vi "BenchmarkToFile.vi"(4 "Memory":dbl, 6 "CPU":dbl, 7 "device name":string, 8 "error in (no error)":errorcluster) -> (0 "error out":errorcluster)   [LabVIEW 2017, in "Benchmarking.lvlib"]
uses:
  <vilib>/addons/InsightCM/Devices/Shared/Common/Benchmarking/Benchmarking.lvlib
  <vilib>/addons/PointValueMap/subVIs/Point_Read_double.vi
  <vilib>/addons/InsightCM/Utilities/GlobalConfiguration/GlobalConfiguration.lvlib
  <vilib>/addons/PointValueMap/PointValueMap.lvlib
  <vilib>/addons/TraceLogger/TraceLogger.lvlib
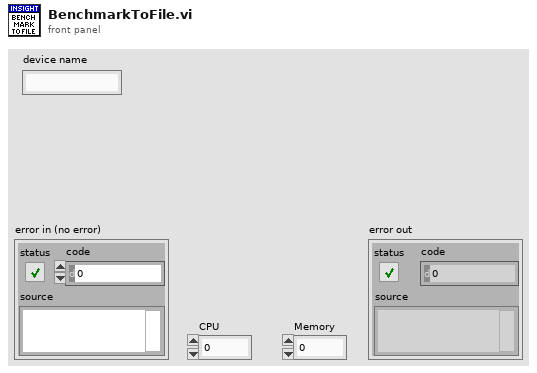
[diagram p1: front panel]
types:
  T1 = enum16{"open", "replace", "create", "open or create", "replace or create", "replace or create with confirmation"}
  T2 = typedef "PointValueMap.lvlib/PointMap.ctl" = refnum<data-value>
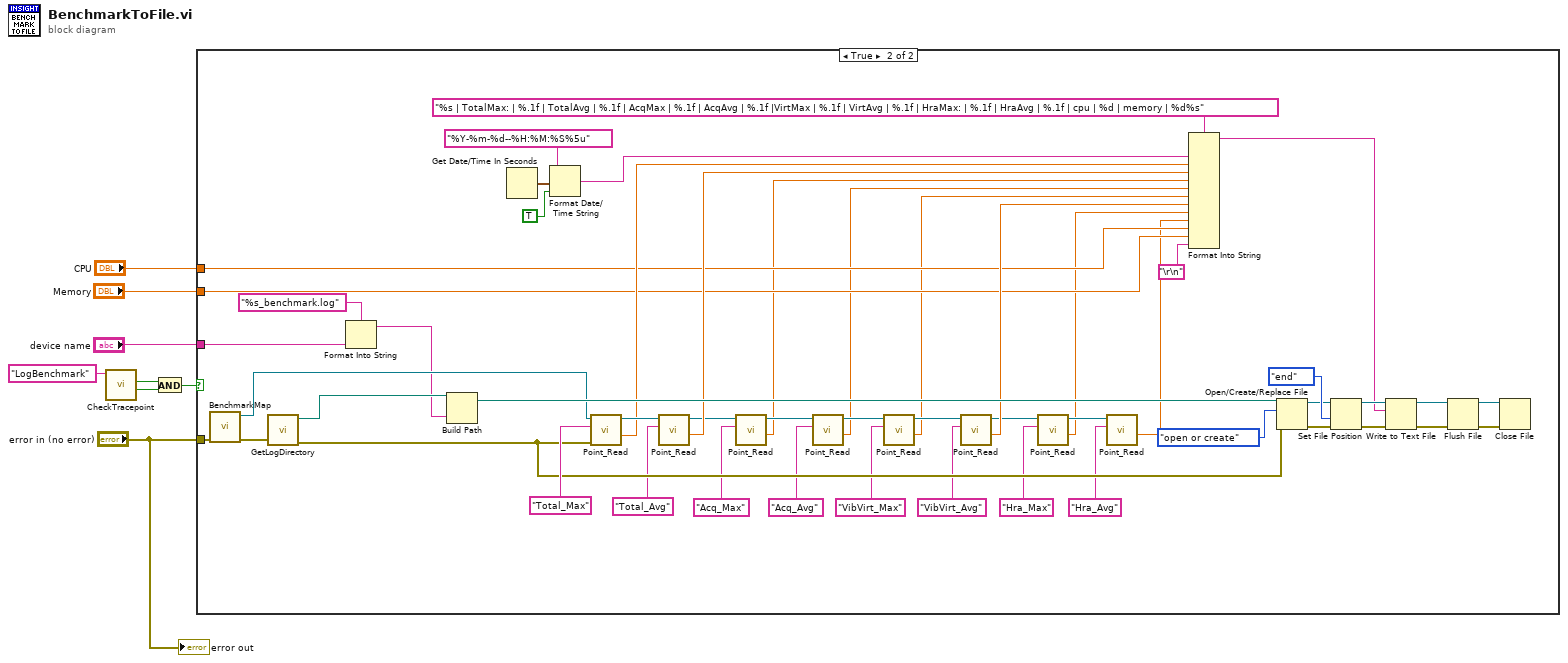
[diagram p0: block diagram]
diagram:
  n1 = call <vilib>:"CheckTracepoint.vi"("tracepoint"="LogBenchmark") -> ("found"=w3:bool, "enabled"=w2:bool)  [unwired: 8 in, 1 out]
  n2 = And(x=w2, y=w3) -> (x .and. y?=w1:bool)
  n3 = case shown="True" w1 {
    tunnel: "CPU" -> [_ w33]
    tunnel: "Memory" -> [_ w32]
    tunnel: "error in (no error)" -> [_ w24]
    tunnel: "device name" -> [_ w21]
    frame False {
    }
    frame True {
      n4 = call <vilib>:"BenchmarkMap.vi"("error in (no error)"=w24) -> ("error out"=w25:errorcluster, "benchmark map"=w23:T2)  [unwired: 9 in]
      n5 = call <vilib>:"GetLogDirectory.vi"("error in (no error)"=w25) -> ("error out"=w42:errorcluster, "log dir"=w44:path)  [unwired: 9 in]
      n6 = Format Into String(format string="%s_benchmark.log", w21) -> (resulting string=w20:string)  [unwired: 2 in, 1 out]
      n7 = Build Path(base path=w44, name or relative path=w20) -> (appended path=w43:path)
      n8 = Get Date/Time In Seconds() -> (seconds since 1Jan1904=w47:timestamp)
      n9 = Format Date/Time String(time format string (%c)="%Y-%m-%d--%H:%M:%S%5u", seconds (now)=w47, UTC format=TRUE) -> (date/time string=w10:string)
      n10 = call-poly <vilib>:"Point_Read.vi"("Error In"=w42, "Tag"="Total_Max", "Map"=w23) -> ("Value"=w38:dbl, "Map Out"=w41:T2)  [unwired: 3 in, 4 out]
      n11 = call-poly <vilib>:"Point_Read.vi"("Tag"="Total_Avg", "Map"=w41) -> ("Value"=w39:dbl, "Map Out"=w16:T2)  [unwired: 4 in, 4 out]
      n12 = call-poly <vilib>:"Point_Read.vi"("Tag"="Acq_Max", "Map"=w16) -> ("Value"=w14:dbl, "Map Out"=w17:T2)  [unwired: 4 in, 4 out]
      n13 = call-poly <vilib>:"Point_Read.vi"("Tag"="Acq_Avg", "Map"=w17) -> ("Value"=w13:dbl, "Map Out"=w15:T2)  [unwired: 4 in, 4 out]
      n14 = call-poly <vilib>:"Point_Read.vi"("Tag"="VibVirt_Max", "Map"=w15) -> ("Value"=w12:dbl, "Map Out"=w37:T2)  [unwired: 4 in, 4 out]
      n15 = call-poly <vilib>:"Point_Read.vi"("Tag"="VibVirt_Avg", "Map"=w37) -> ("Value"=w34:dbl, "Map Out"=w31:T2)  [unwired: 4 in, 4 out]
      n16 = call-poly <vilib>:"Point_Read.vi"("Tag"="Hra_Max", "Map"=w31) -> ("Value"=w27:dbl, "Map Out"=w30:T2)  [unwired: 4 in, 4 out]
      n17 = call-poly <vilib>:"Point_Read.vi"("Tag"="Hra_Avg", "Map"=w30) -> ("Value"=w26:dbl)  [unwired: 4 in, 5 out]
      n18 = Format Into String(format string="%s | TotalMax: | %.1f | TotalAvg | %.1f | AcqMax | %.1f | AcqAvg | %.1f |VirtMax | %.1f | VirtAvg | %.1f | HraMax: | %.1f | HraAvg | %.1f | cpu | %d | memory | %d%s", w10, w38, w39, w14, w13, w12, w34, w27, w26, w33, w32, "\r\n") -> (resulting string=w11:string)  [unwired: 2 in, 1 out]
      n19 = Open/Create/Replace File(file path (use dialog)=w43, error in=w42, operation (0:open)=T1."open or create") -> (refnum out=w55:refnum<file>, error out=w56:errorcluster)  [unwired: 3 in, 1 out]
      n20 = Set File Position(refnum=w55, from (0:start)=enum16{"start", "end", "current"}."end", error in=w56) -> (refnum out=w58:refnum<file>, error out=w59:errorcluster)  [unwired: 1 in]
      n21 = Write to Text File(file (use dialog)=w58, text=w11, error in=w59) -> (refnum out=w51:refnum<file>, error out=w52:errorcluster)  [unwired: 1 in, 1 out]
      n22 = Flush File(refnum=w51, error in=w52) -> (refnum out=w50:refnum<file>, error out=w53:errorcluster)
      n23 = Close File(refnum=w50, error in=w53) -> ()  [unwired: 2 out]
    }
  }
  "error out" <- "error in (no error)"
